vi "passTestResult.vi"(11 "State":T1=enum."Pass intercepted") -> (3 "Pass state":T1)   [LabVIEW 2017]
uses:
  passTestStates.ctl
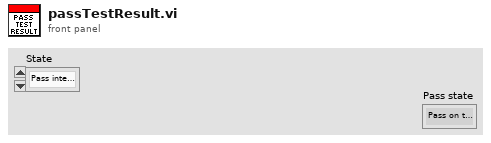
[diagram p1: front panel]
types:
  T1 = typedef "passTestStates.ctl" = enum16{"Pass on the way", "Ball stops", "Pass intercepted", "Ball out of the field", "Ball missed robot", "Need more force to pass", "Too much force", "Correct pass", "Keep ball possesion", "Robot kicked the ball", "Waiting Kick", "Invalid: same robot", "Invalid: kicker ID 999", "Invalid: Receiver ID 999", "Invalid"}
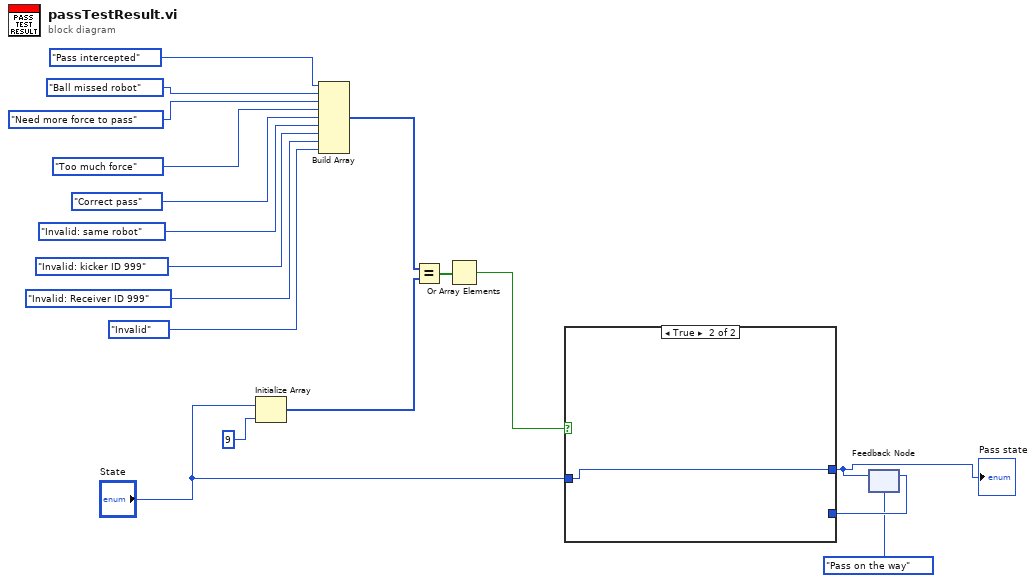
[diagram p0: block diagram]
diagram:
  n1 = Initialize Array("State", 9 ("dimension size")) -> (w7:T1[])
  n2 = Build Array(passTestStates."Pass intercepted" ("Result"), passTestStates."Ball missed robot" ("Result"), passTestStates."Need more force to pass" ("Result"), passTestStates."Too much force" ("Result"), passTestStates."Correct pass" ("Result"), passTestStates."Invalid: same robot" ("Result"), passTestStates."Invalid: kicker ID 999" ("Result"), passTestStates."Invalid: Receiver ID 999" ("Result"), passTestStates."Invalid" ("Result")) -> (w8:T1[])
  n3 = Equal?(x=w8, y=w7) -> (x = y?=w6:bool[])
  n4 = Or Array Elements(Boolean array=w6) -> (logical OR=w4:bool)
  n5 = feedback #1(passTestStates."Pass on the way" ("State")) -> (w2:T1)
  n6 = case shown="True" w4 {
    tunnel: "State" -> [_ w20]
    tunnel: [w19 w20] -> w3
    tunnel: w2 -> [w19 _]
    frame False {
    }
    frame True {
    }
  }
  "Pass state" <- w3
  n7 = feedback-in #1(w3) -> ()
